vi "vi_get_callees.vi"(8 "error in (no error)":errorcluster, 10 "VINode":refnum<class "HierarchyNode.lvclass">, 11 "VIGraph in":refnum<class "HierarchyGraph.lvclass">) -> (0 "error out":errorcluster, 2 "Callees":refnum<class "HierarchyNode.lvclass">[](array[class]))   [LabVIEW 2020, in "vi-hierarchy.lvlib" / "HierarchyGraph.lvclass"]
uses:
  HierarchyGraph.lvclass
  VINode/HierarchyNode.lvclass
  Y:/FlowRails/lv-graph/source/api/Node/Node.lvclass
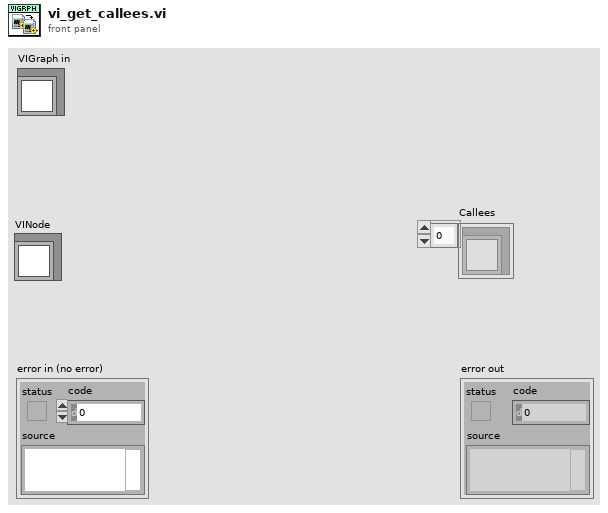
[diagram p1: front panel]
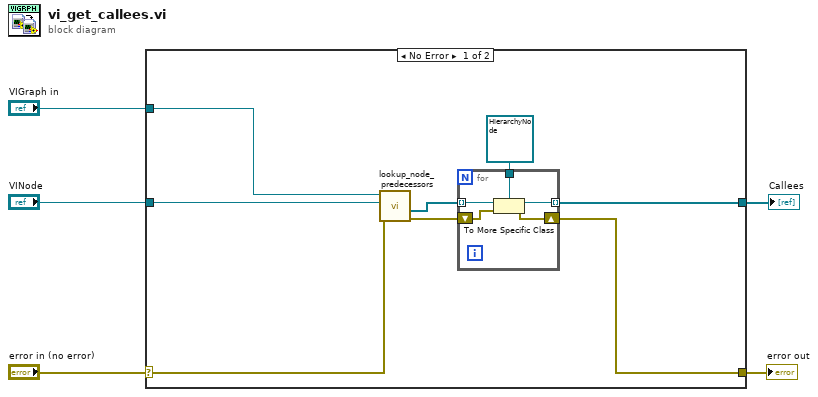
[diagram p0: block diagram]
diagram:
  n1 = case shown="No Error" "error in (no error)" {
    selector: "error in (no error)" -> [w12 w19]
    tunnel: [w8 w19] -> w4
    tunnel: "VIGraph in" -> [w13 _]
    tunnel: "VINode" -> [w11 _]
    tunnel: [w10 _] -> w1
    frame No Error {
      n2 = call-dynamic "lookup_node_predecessors.vi"("error in (no error)"=w12, "node"=w11, "digraph"=w13) -> ("error out"=w9:errorcluster, "predecessors"=w6:refnum<class "Node.lvclass">[])  [unwired: 7 in]
      n3 = for {
        tunnel: w6 -> [w18] mode=indexing
        tunnel: [w17] -> w10 mode=indexing
        tunnel: refnum<class "HierarchyNode.lvclass"> refnum ("VINode") -> [w14]
        shift-right: [w15] -> w8
        shift-left: w9 -> [w16]
        n4 = To More Specific Class(target class=w14, reference=w18, error in=w16) -> (specific class reference=w17:refnum<class "HierarchyNode.lvclass">, error out=w15:errorcluster)
      }
    }
    frame Error {
    }
  }
  "error out" <- w4
  "Callees" <- w1
